vi "PH_VacuumControl.PC Set Logarithmic.vi"(0 "i ref in":refnum<vi>, 2 "Logarithmic":bool, 5 "error IO":errorcluster) -> (14 "i ref out":refnum<vi>, 19 "error out":errorcluster)   [LabVIEW 2014, in "PH_VacuumControl.lvlib"]
doc: "This VI sets the Trend GUI element to logarithmic scale."
uses:
  PH_VacuumControl.lvlib
  PH_Basics/PH_Common/PH_Common.lvlib
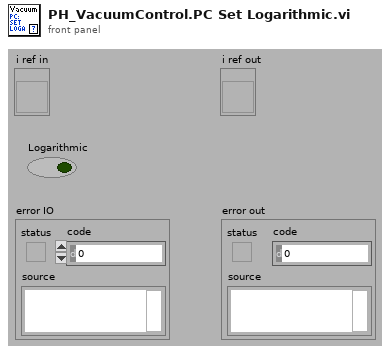
[diagram p1: front panel]
types:
  T1 = typedef "PH_VacuumControl.lvlib/PH_VacuumControl.i attribute.ctl" = cluster{"GUI Refs":cluster{"Exit":refnum<vi>, "Set Unit":refnum<vi>, "Device found":refnum<vi>, "Busy":refnum<vi>, "State":refnum<vi>, "Delete":refnum<vi>, "Channels":refnum<vi>, "Channel Name":refnum<vi>, "Trend":refnum<vi>, "Logarithmic":refnum<vi>, "Limit reached":refnum<vi>, "Channel Name 1 MT":refnum<vi>, "Channel Name 2 MT":refnum<vi>, "Trend MT":refnum<vi>, "Logarithmic MT":refnum<vi>, "Limit reached MT":refnum<vi>}, "Device found":bool, "Busy":bool, "Selected Unit":i32, "Channels [mbar]":T2, "Channel Names":cluster{"Channel 1":string, "Channel 2":string, "Channel 3":string, "Channel 4":string, "Channel 5":string, "Channel 6":string}, "Status":T3, "AGCxxx VISA Cluster":T4, "Instr Firmware Revision":string, "Service IDs Pressure":cluster{"Channel 1":i32, "Channel 2":i32, "Channel 3":i32, "Channel 4":i32, "Channel 5":i32, "Channel 6":i32}, "Service IDs Limits":cluster{"Channel 1":i32, "Channel 2":i32, "Channel 3":i32, "Channel 4":i32, "Channel 5":i32, "Channel 6":i32}, "Trend":cluster{"Start Point":timestamp, "Pressures [mbar] Channel 1":dbl[], "Pressures [mbar] Channel 2":dbl[], "Pressures [mbar] Channel 3":dbl[], "Pressures [mbar] Channel 4":dbl[], "Pressures [mbar] Channel 5":dbl[], "Pressures [mbar] Channel 6":dbl[], "Timebase [s]":i32[], "Trend Channel":u16, "Start Fit":dbl, "Trend Channel 1 MT":u16, "Trend Channel 2 MT":u16, "Start or continue Fit MT":dbl, "Continue or start Fit MT":dbl, "Datasets strored":i32, "Dataarray Size":i32}, "Running":bool}
  T2 = typedef "PH_VacuumControl.lvlib/PH_VacuumControl.Channels.ctl" = cluster{"Channel 1":dbl, "Channel 2":dbl, "Channel 3":dbl, "Channel 4":dbl, "Channel 5":dbl, "Channel 6":dbl, "Name Channel 1":string, "Name Channel 2":string, "Name Channel 3":string, "Name Channel 4":string, "Name Channel 5":string, "Name Channel 6":string, "Upper Limit":dbl, "Upper Limit 2":dbl, "Upper Limit 3":dbl, "Upper Limit 4":dbl, "Upper Limit 5":dbl, "Upper Limit 6":dbl}
  T3 = typedef "PH_StatusHandler.lvlib/PH_StatusHandler.Status.ctl" = i16
  T4 = typedef "AGCxxx - Driver.lvlib/AGCxxx VISA Control.ctl" = cluster{"VISA resource name":refnum<visa-resource-name>, "VISA Timeout Value (1000 ms)":u32, "Lock Timeout (1000 ms)":u32, "MAX Channel (6)":i32}
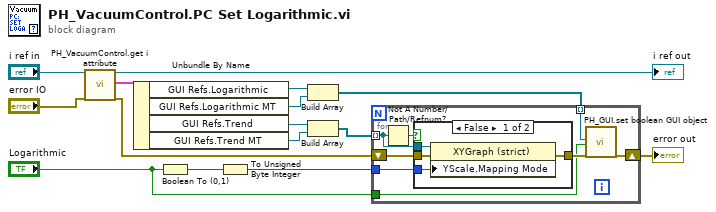
[diagram p0: block diagram]
diagram:
  n1 = call "PH_VacuumControl.get i attribute.vi"("i ref in"="i ref in", "error in (no error)"="error IO") -> ("i ref out"=→"i ref out":refnum<vi>, "i attribute"=w11:T1, "error out"=w12:errorcluster)  [unwired: 15 in]
  n2 = Unbundle By Name(w11) -> ("GUI Refs.Logarithmic"=w15:refnum<vi>, "GUI Refs.Logarithmic MT"=w3:refnum<vi>, "GUI Refs.Trend"=w13:refnum<vi>, "GUI Refs.Trend MT"=w1:refnum<vi>)
  n3 = Boolean To (0,1)(Boolean="Logarithmic") -> (0, 1=w6:i16)
  n4 = To Unsigned Byte Integer(number=w6) -> (unsigned 8bit integer=w5:u8)
  n5 = Build Array(w15, w3) -> (w4:refnum<vi>[])
  n6 = Build Array(w13, w1) -> (w2:refnum<vi>[])
  n7 = for {
    tunnel: w4 -> [w23] mode=indexing
    tunnel: w2 -> [w19] mode=indexing
    tunnel: "Logarithmic" -> [w17]
    tunnel: w5 -> [w16]
    shift-right: [w21] -> w14
    shift-left: w12 -> [w18]
    n8 = Not A Number/Path/Refnum?(number/path/refnum=w19) -> (NaN/Path/Refnum?=w20:bool)
    n9 = case shown="False" w20 {
      tunnel: w16 -> [w27 _]
      tunnel: w19 -> [w26 _]
      tunnel: w18 -> [w25 w28]
      tunnel: [w24 w28] -> w22
      frame False {
        n10 = property class="XYGraph (strict)"(reference=w26, error in=w25, "YScale.Mapping Mode"=w27) -> (error out=w24:errorcluster)  [unwired: 1 out]
      }
      frame True {
      }
    }
    n11 = call "PH_GUI.set boolean GUI object.vi"("Boolean Knob GUI Ref"=w23, "Value"=w17, "error in (no error)"=w22) -> ("error out"=w21:errorcluster)  [unwired: 16 in]
  }
  "error out" <- w14
